vi "Handle Missing Sections.vi"(5 "section (optional)":string, 6 "any found?":bool, 7 "Section Formatted Cluster In":variant, 8 "error in (no error)":errorcluster, 9 "all found?":bool, 10 "Section Formatted Cluster in":variant, 11 "Refnum in":T1) -> (0 "error out":errorcluster, 2 "Section Formatted Cluster out":variant, 3 "Refnum out":T1)   [LabVIEW 2019, in "Configuration.lvclass"]
uses:
  Configuration.lvclass
  <vilib>/Utility/config.llb/Config Data RefNum.ctl
  <vilib>/Utility/config.llb/NI_LVConfig.lvlib
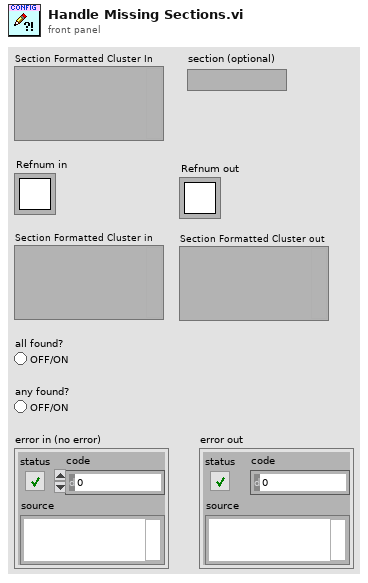
[diagram p1: front panel]
types:
  T1 = typedef "NI_LVConfig.lvlib/Config Data RefNum.ctl" = refnum<k1>
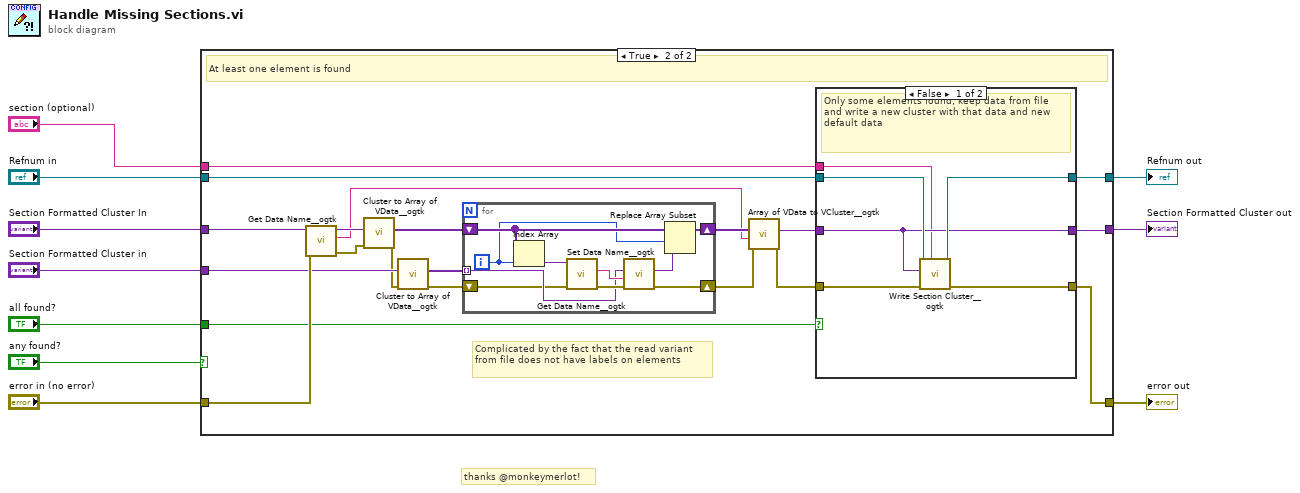
[diagram p0: block diagram]
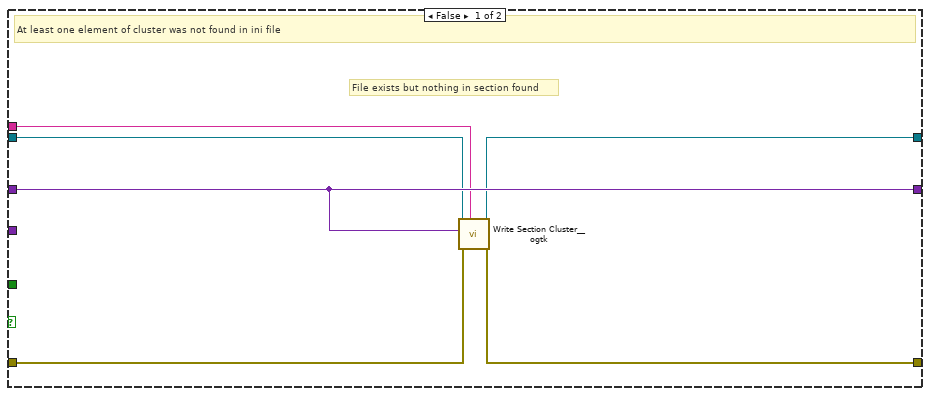
[diagram p2: hidden frame]
diagram:
  # "thanks @monkeymerlot!"
  n1 = case shown="True" "any found?" {
    tunnel: "Section Formatted Cluster In" -> [w16 w34]
    tunnel: "Section Formatted Cluster in" -> [_ w35]
    tunnel: "Refnum in" -> [w12 w19]
    tunnel: [w13 w20] -> w6
    tunnel: [w16 w22] -> w7
    tunnel: "error in (no error)" -> [w15 w36]
    tunnel: [w14 w23] -> w9
    tunnel: "all found?" -> [_ w24]
    tunnel: "section (optional)" -> [w11 w17]
    frame False {
      # "File exists but nothing in section found"
      # "At least one element of cluster was not found in ini file"
      n2 = call <userlib>:"Write Section Cluster__ogtk.vi"("section (optional)"=w11, "error in (no error)"=w15, "Section Formatted Cluster"=w16, "refnum"=w12) -> ("error out"=w14:errorcluster, "dup refnum"=w13:T1)  [unwired: 6 in]
    }
    frame True {
      # "Complicated by the fact that the read variant from file does not have labels on elements"
      # "At least one element is found"
      n3 = call <userlib>:"Get Data Name__ogtk.vi"("error in (no error)"=w36, "Data"=w34) -> ("error out"=w27:errorcluster, "Data Name"=w28:string, "Data dup"=w29:variant)  [unwired: 7 in]
      n4 = call <userlib>:"Cluster to Array of VData__ogtk.vi"("error in (no error)"=w27, "Cluster"=w29) -> ("error out"=w33:errorcluster, "Array of VData"=w32:variant[])  [unwired: 8 in]
      n5 = call <userlib>:"Cluster to Array of VData__ogtk.vi"("error in (no error)"=w33, "Cluster"=w35) -> ("error out"=w26:errorcluster, "Array of VData"=w31:variant[])  [unwired: 8 in]
      n6 = for {
        tunnel: w31 -> [w39] mode=indexing
        shift-right: [w46] -> w30
        shift-left: w32 -> [w45]
        shift-right: [w37] -> w25
        shift-left: w26 -> [w38]
        i -> [w44]
        n7 = Index Array(array=w45, index=w44) -> (element=w43:variant)
        n8 = call <userlib>:"Get Data Name__ogtk.vi"("error in (no error)"=w38, "Data"=w43) -> ("error out"=w40:errorcluster, "Data Name"=w41:string)  [unwired: 7 in, 1 out]
        n9 = call <userlib>:"Set Data Name__ogtk.vi"("error in (no error)"=w40, "Data Name"=w41, "Data"=w39) -> ("error out"=w37:errorcluster, "Renamed Data"=w42:variant)  [unwired: 7 in]
        n10 = Replace Array Subset(array=w45, new element=w42, index=w44) -> (w46:variant[])
      }
      n11 = call <userlib>:"Array of VData to VCluster__ogtk.vi"("error in (no error)"=w25, "Cluster Name"=w28, "Array"=w30) -> ("error out"=w18:errorcluster, "VCluster"=w21:variant)  [unwired: 7 in]
      n12 = case shown="False" w24 {
        tunnel: w18 -> [w49 w55]
        tunnel: [w50 w55] -> w23
        tunnel: [w48 w54] -> w22
        tunnel: w21 -> [w48 w54]
        tunnel: w19 -> [w52 w53]
        tunnel: [w51 w53] -> w20
        tunnel: w17 -> [w47 _]
        frame False {
          # "Only some elements found, keep data from file and write a new cluster with that data and new default data"
          n13 = call <userlib>:"Write Section Cluster__ogtk.vi"("section (optional)"=w47, "error in (no error)"=w49, "Section Formatted Cluster"=w48, "refnum"=w52) -> ("error out"=w50:errorcluster, "dup refnum"=w51:T1)  [unwired: 6 in]
        }
        frame True {
          # "all elements found"
        }
      }
    }
  }
  "error out" <- w9
  "Section Formatted Cluster out" <- w7
  "Refnum out" <- w6
